vi "close.vi"(8 "error in":errorcluster, 11 "dds runtime in":refnum<class "DDS runtime.lvclass">) -> (0 "error out":errorcluster)   [LabVIEW 2013, in "DDS runtime.lvclass"]
doc: "Provides an interface for terminating a module instance. While this interface performs no operations, a child should close and deallocate any open references or memory."
uses:
  DDS runtime.lvclass
  DDS runtime.lvclass/DDS runtime.ctl
  <vilib>/RTI DDS Toolkit for LabVIEW/Library/LVDDS_library.lvlib
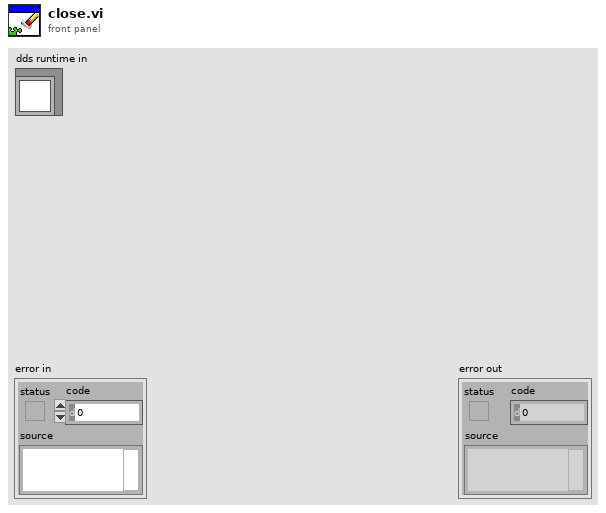
[diagram p1: front panel]
types:
  T1 = typedef "tag bus.lvlib/tag descriptor.lvclass/Data Type.ctl" = enum16{"Double", "Single", "I64", "I32", "I16", "I8", "U64", "U32", "U16", "U8", "Boolean", "String", "Array of Double", "Array of Single", "Array of I64", "Array of I32", "Array of I16", "Array of I8", "Array of U64", "Array of U32", "Array of U16", "Array of U8", "Array of Boolean", "Array of String"}
  T2 = cluster{"index":i32, "data type":T1, "ref num":u64, "new samples only":bool, "query condition":string}[]
  T3 = cluster{"index":i32, "data type":T1, "ref num":u64}[]
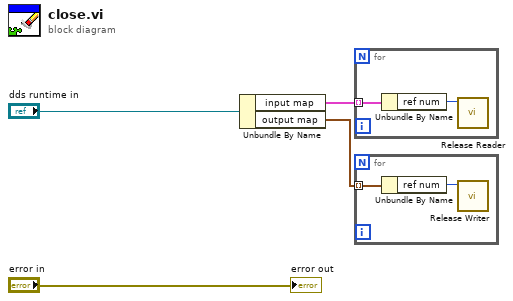
[diagram p0: block diagram]
diagram:
  n1 = Unbundle By Name("dds runtime in") -> ("input map"=w2:T2, "output map"=w1:T3)
  n2 = for {
    tunnel: w2 -> [w6] mode=indexing
    n3 = Unbundle By Name(w6) -> ("ref num"=w5:u64)
    n4 = call <vilib>:"Release Reader.vi"("ref num"=w5) -> ()  [unwired: 10 in, 1 out]
  }
  n5 = for {
    tunnel: w1 -> [w8] mode=indexing
    n6 = Unbundle By Name(w8) -> ("ref num"=w7:u64)
    n7 = call <vilib>:"Release Writer.vi"("ref num"=w7) -> ()  [unwired: 10 in, 1 out]
  }
  "error out" <- "error in"
